vi "Fin_status.vi"(8 "Error In":errorcluster, 10 "Round Color Box":u32, 11 "Fin Index":i32) -> (0 "Error Out":errorcluster)   [LabVIEW 2013]
uses:
  My Computer/Controls/Fin Status.ctl
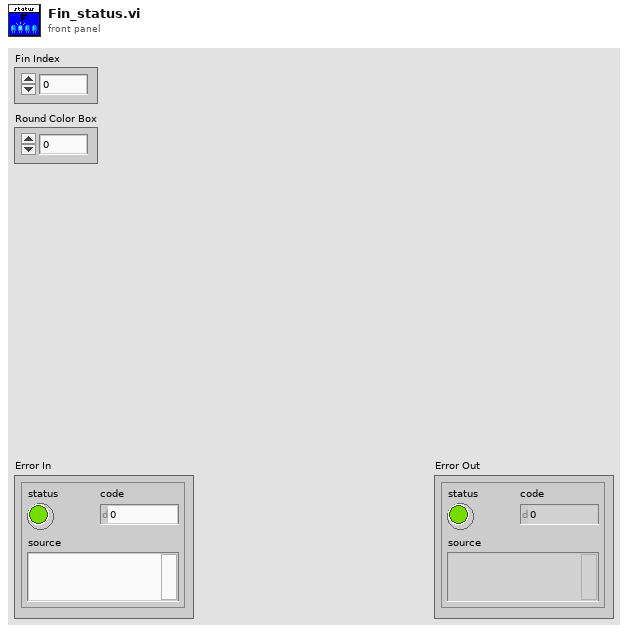
[diagram p1: front panel]
types:
  T1 = typedef "Fin Status.ctl" = u32[]
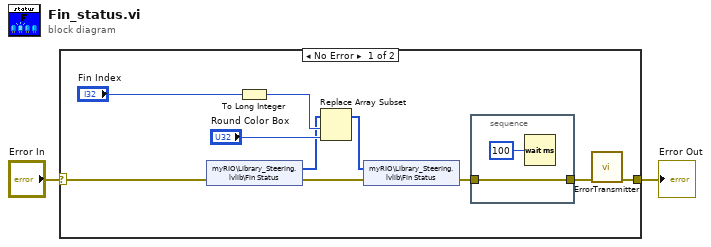
[diagram p0: block diagram]
diagram:
  n1 = case shown="No Error" "Error In" {
    selector: "Error In" -> [w5 w15]
    tunnel: [w3 w15] -> w2
    frame No Error {
      n2 = shared-variable "myRIO\\Library_Steering.lvlib\\Fin Status"(error in=w5) -> (w7:T1, error out=w9:errorcluster)
      n3 = To Long Integer(number="Fin Index") -> (32bit integer=w10:i32)
      n4 = Replace Array Subset(array=w7, new element="Round Color Box", index=w10) -> (w8:T1)
      n5 = shared-variable "myRIO\\Library_Steering.lvlib\\Fin Status"(w8, error in=w9) -> (error out=w6:errorcluster)
      n6 = stacked-sequence {
        tunnel: w6 -> [w13]
        tunnel: [w13] -> w4
        frame #0 {
          n7 = Wait (ms)(milliseconds to wait=u32 100) -> ()  [unwired: 1 out]
        }
      }
      n8 = call "ErrorTransmitter.vi"("Error In"=w4) -> ("Error Out"=w3:errorcluster)  [unwired: 10 in]
    }
    frame Error {
    }
  }
  "Error Out" <- w2
